vi "ExecPratAulaWhileFC.vi"() -> ()   [LabVIEW 2020]
panel:
  in  "Boolean":bool
  out "Celsius":dbl(slide) scale=-200.0..100.0
  in  "Farhenreit":dbl(slide) scale=0.0..300.0
  in  "milliseconds to wait":u32
  out "(i)":i32
  in  "stop":bool
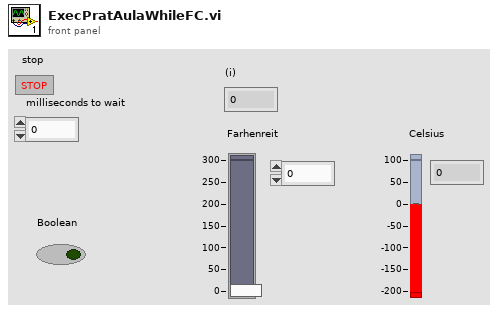
[diagram p1: front panel]
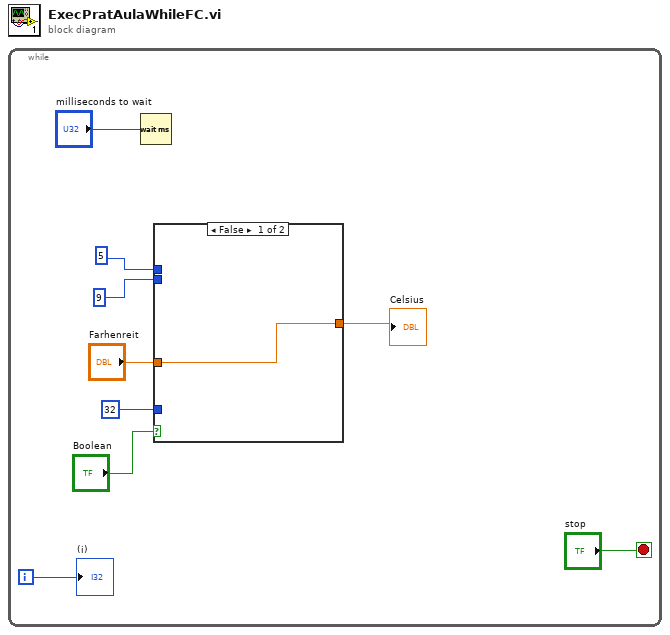
[diagram p0: block diagram]
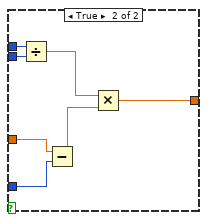
[diagram p2: hidden frame]
diagram:
  n1 = while {
    i -> [w8]
    stop <- "stop" stop-if-true
    n2 = Wait (ms)(milliseconds to wait="milliseconds to wait") -> ()  [unwired: 1 out]
    n3 = case shown="False" "Boolean" {
      tunnel: 5 -> [_ w17]
      tunnel: 9 -> [_ w16]
      tunnel: "Farhenreit" -> [w10 w15]
      tunnel: 32 -> [_ w14]
      tunnel: [w10 w11] -> w2
      frame False {
      }
      frame True {
        n4 = Divide(x=w17, y=w16) -> (x/y=w13:dbl)
        n5 = Subtract(x=w15, y=w14) -> (x-y=w12:dbl)
        n6 = Multiply(x=w13, y=w12) -> (x*y=w11:dbl)
      }
    }
    "Celsius" <- w2
    "(i)" <- w8
  }
